vi "New.vi"(8 "error in (no error)":errorcluster, 9 "UE:From1PLOT":refnum<user-event>, 10 "Type":T5, 11 "ChannelMap":map{string, T1}(c390)) -> (0 "error out":errorcluster, 2 "callback UEs":T4, 3 "StokePlotHandle out":refnum<class "BjusticePlotHandle.lvclass">)   [LabVIEW 2021, in "BjusticePlotHandle.lvclass"]
uses:
  BjusticePlotHandle.lvclass
  Type.ctl
  1PLOT to MPLOT UE.ctl
  1PLOT to MPLOT type.ctl
  <userlib>/bjustice/Ring Buffer for Time Series Data Strict Accessor/SubVIs/RingBufferHandle.ctl
  <userlib>/bjustice/Ring Buffer for Time Series Data/SubVIs/DVR data.ctl
  <userlib>/bjustice/Ring Buffer for Time Series Data Strict Accessor/SubVIs/DataType.ctl
  <userlib>/bjustice/Ring Buffer for Time Series Data Strict Accessor/SubVIs/Endianess.ctl
  BjusticePlotHandle.lvclass/BjusticePlotHandle.ctl
  <userlib>/bjustice/Ring Buffer for Time Series Data/Ring Buffer Time Series Data.lvlib
  <userlib>/bjustice/Ring Buffer for Time Series Data Strict Accessor/Ring Buffer Strict Accessor.lvlib
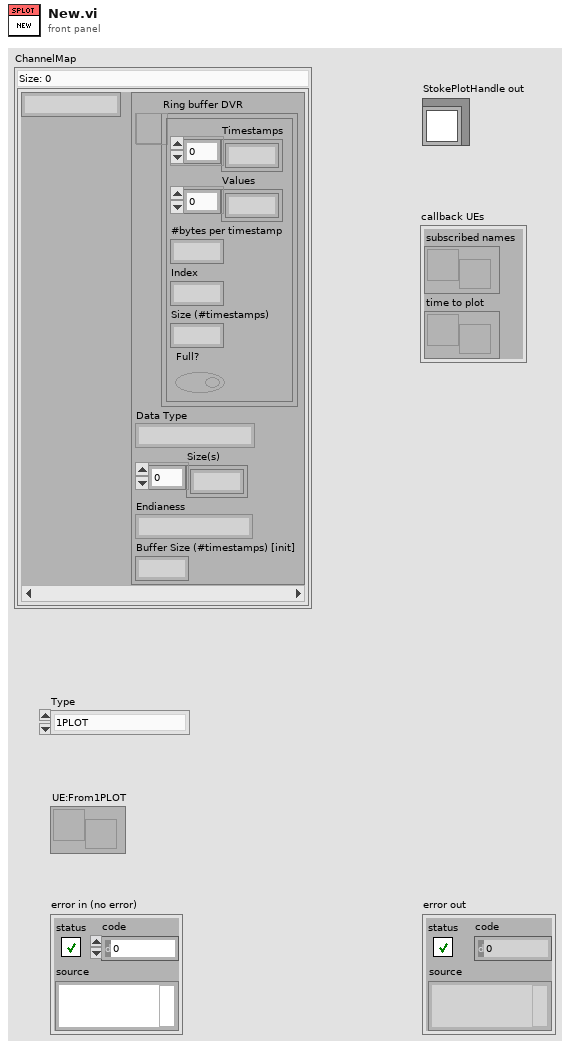
[diagram p1: front panel]
types:
  T1 = typedef "Ring Buffer Strict Accessor.lvlib/RingBufferHandle.ctl" = cluster{"Ring buffer DVR":refnum<data-value>, "Data Type":T2, "Size(s)":i32[], "Endianess":T3, "Buffer Size (#timestamps) [init]":i32}
  T2 = typedef "Ring Buffer Strict Accessor.lvlib/DataType.ctl" = enum16{"uint8", "uint16", "uint32", "uint64", "int8", "int16", "int32", "int64", "float", "double", "extended"}
  T3 = typedef "Ring Buffer Strict Accessor.lvlib/Endianess.ctl" = enum16{"big-endian", "little-endian"}
  T4 = cluster{"subscribed names":refnum<user-event>, "time to plot":refnum<user-event>}
  T5 = typedef "BjusticePlotHandle.lvclass/Type.ctl" = enum16{"1PLOT", "MPLOT"}
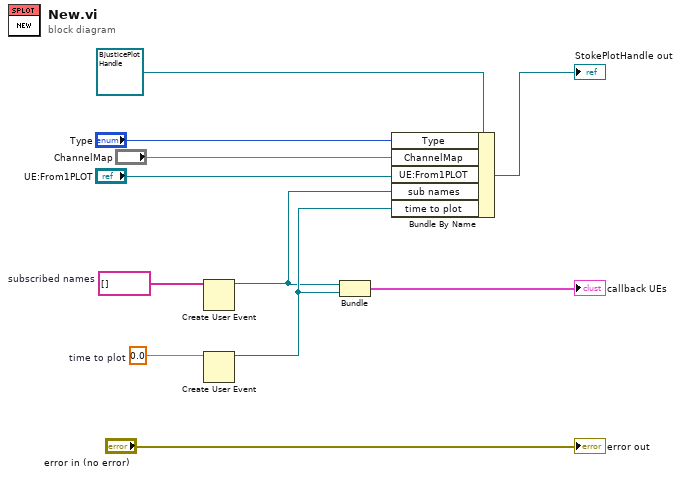
[diagram p0: block diagram]
diagram:
  w5 = 0.0  # time to plot
  w6 = string[] []  # subscribed names
  n1 = Create User Event(user event datatype=w6) -> (user event=w2:refnum<user-event>)  [unwired: 1 in, 1 out]
  n2 = Create User Event(user event datatype=w5) -> (user event=w3:refnum<user-event>)  [unwired: 1 in, 1 out]
  n3 = Bundle("subscribed names"=w2, "time to plot"=w3) -> (→"callback UEs":T4)  [unwired: 1 in]
  n4 = Bundle By Name(cluster=refnum<class "BjusticePlotHandle.lvclass"> refnum ("StokePlotHandle out"), "Type"="Type", "ChannelMap"="ChannelMap", "UE:From1PLOT"="UE:From1PLOT", "sub names"=w2, "time to plot"=w3) -> (→"StokePlotHandle out":refnum<class "BjusticePlotHandle.lvclass">)
  "error out" <- "error in (no error)"
